vi "Init Events.vi"(8 "error in (no error)":errorcluster, 11 "DeviceDetailPanel in":refnum<class "DeviceDetailPanel.lvclass">) -> (0 "error out":errorcluster, 3 "DeviceDetailPanel out":refnum<class "DeviceDetailPanel.lvclass">)   [LabVIEW 2020, in "PicoG-App.lvlib" / "DeviceDetailPanel.lvclass"]
uses:
  DeviceDetailPanel.lvclass
  DeviceDetailPanel.lvclass/DeviceDetailPanel.ctl
  ViaApp/ViaApp.lvclass
  Device/Device.lvclass
  Deploy Data.ctl
  PicoG-App.lvlib
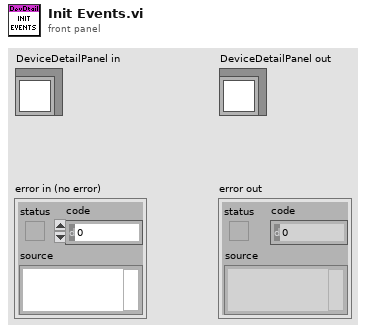
[diagram p1: front panel]
types:
  T1 = typedef "PicoG-App.lvlib/Deploy Data.ctl" = cluster{"App":refnum<class "ViaApp.lvclass">, "Device":refnum<class "Device.lvclass">}
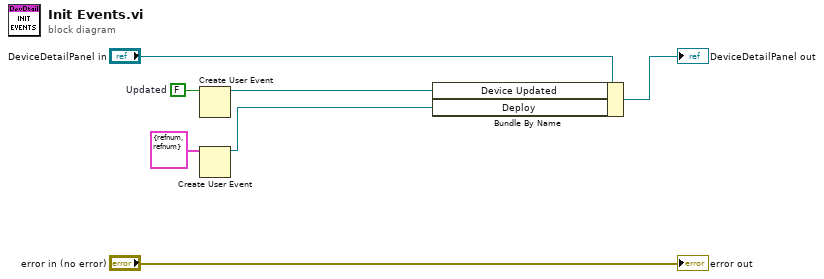
[diagram p0: block diagram]
diagram:
  w4 = FALSE  # Updated
  n1 = Create User Event(user event datatype=w4) -> (user event=w3:refnum<user-event>)  [unwired: 1 in, 1 out]
  n2 = Create User Event(user event datatype=T1 {"App"=refnum, "Device"=refnum} ("Deploy Data")) -> (user event=w1:refnum<user-event>)  [unwired: 1 in, 1 out]
  n3 = Bundle By Name(cluster="DeviceDetailPanel in", "Device Updated"=w3, "Deploy"=w1) -> (→"DeviceDetailPanel out":refnum<class "DeviceDetailPanel.lvclass">)
  "error out" <- "error in (no error)"
